vi "CRYAlignment Harmonic Orders.vi"(10 "Harmonics Orders In":dbl[](array[numeric]), 11 "HT Option":bool[](array[boolean])) -> (3 "Harmonics Orders Out":dbl[](array[numeric]))   [LabVIEW 2013]
panel:
  # "* measurement confidence\n0. Standard Error\n1. Confidence Limits\n2. Total Noise\n\n*Harmonics\n3. Harmonics @meas.Frq\n4. Total Distortion\n5. THD [%]\n6. THD Normalized [%]\n7. THD + Noise [%]\n8. Rub & Buzz [%]\n9. Rub & Buzz Norm'd [%]\n\nIM\n10. Total IM\n11. Total IM [%]\n12. Total IM + Noise [%]\n\nDiff\n13. Total Diff\n14. Total DFD [%]\n15. Total DFD + Noise [%]"
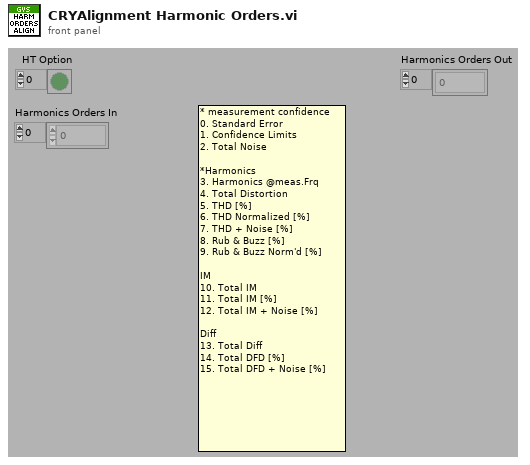
[diagram p1: front panel]
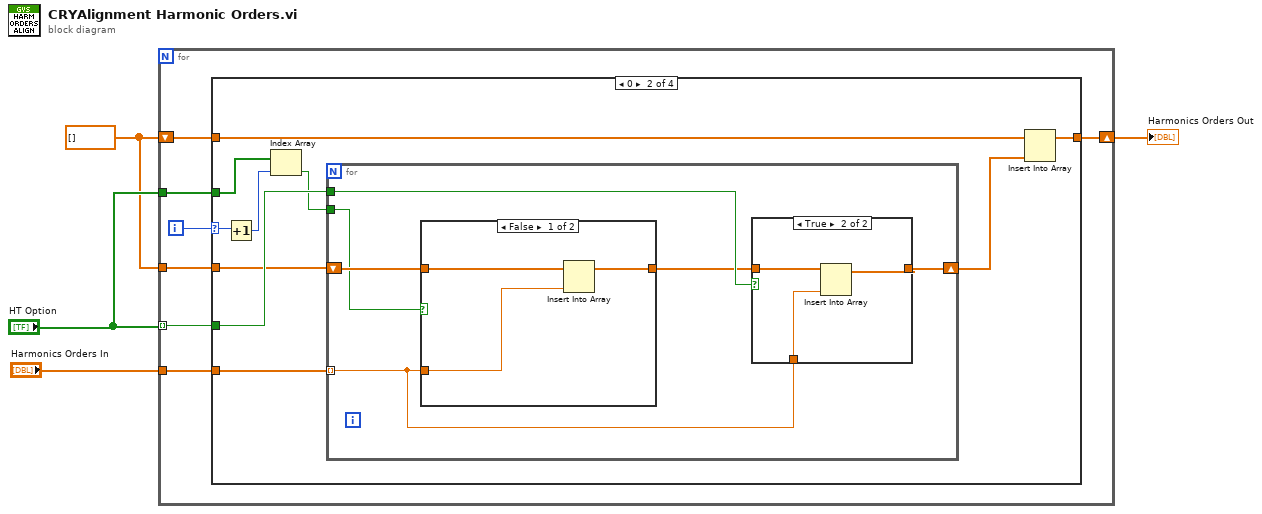
[diagram p0: block diagram]
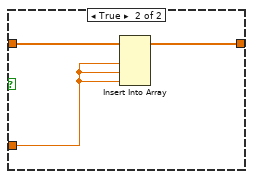
[diagram p4: hidden frame]
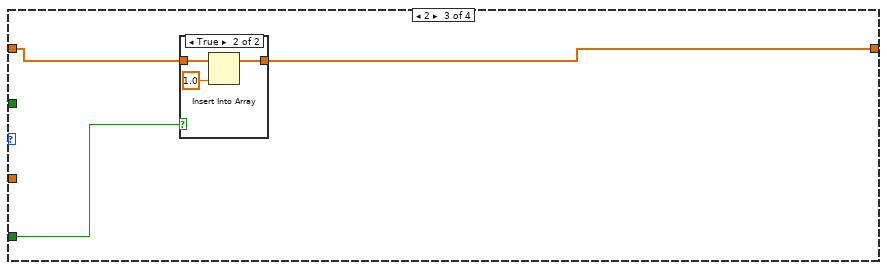
[diagram p5: hidden frame]
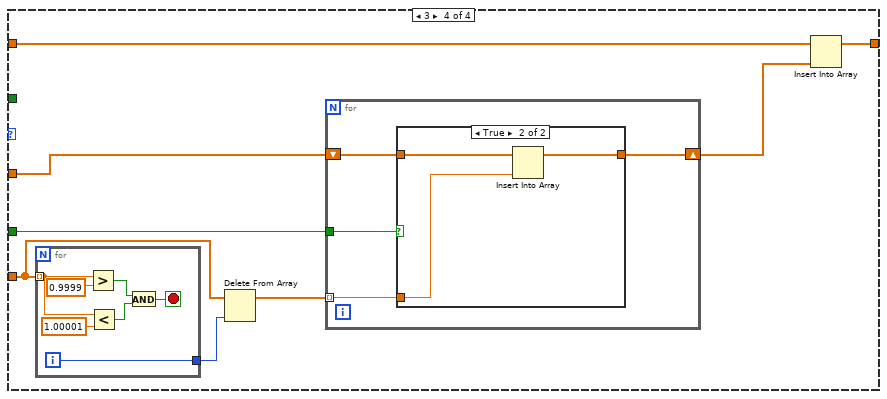
[diagram p7: hidden frame]
diagram:
  w2 = dbl[] [] ("Harmonics Orders")
  n1 = for {
    tunnel: "HT Option" -> [w9] mode=indexing
    shift-right: [w10] -> w1
    shift-left: w2 -> [w11]
    tunnel: "HT Option" -> [w7]
    tunnel: w2 -> [w6]
    tunnel: "Harmonics Orders In" -> [w5]
    i -> [w8]
    n2 = case shown="0" w8 {
      selector: w8 -> [_ w20 _ _]
      tunnel: w11 -> [w12 w16 w41 w48]
      tunnel: [w12 w17 w40 w47] -> w10
      tunnel: w9 -> [_ w22 w39 w53]
      tunnel: w7 -> [_ w21 _ _]
      tunnel: w6 -> [_ w14 _ w50]
      tunnel: w5 -> [_ w13 _ w51]
      frame Default {
      }
      frame 0 {
        n3 = Increment(x=w20) -> (x+1=w19:i32)
        n4 = Index Array(array=w21, index=w19) -> (element=w18:bool)
        n5 = for {
          tunnel: w18 -> [w26]
          shift-right: [w27] -> w15
          shift-left: w14 -> [w28]
          tunnel: w22 -> [w25]
          tunnel: w13 -> [w23] mode=indexing
          n6 = case shown="False" w26 {
            tunnel: w28 -> [w35 w38]
            tunnel: [w34 w37] -> w24
            tunnel: w23 -> [w33 w36]
            frame False {
              n7 = Insert Into Array(array=w35, new element=w33) -> (w34:dbl[])  [unwired: 1 in]
            }
            frame True {
              n8 = Insert Into Array(array=w38, new element #1=w36, new element #2=w36, new element #3=w36) -> (w37:dbl[])  [unwired: 1 in]
            }
          }
          n9 = case shown="True" w25 {
            tunnel: w24 -> [w29 w32]
            tunnel: [w29 w31] -> w27
            tunnel: w23 -> [_ w30]
            frame False {
            }
            frame True {
              n10 = Insert Into Array(array=w32, new element=w30) -> (w31:dbl[])  [unwired: 1 in]
            }
          }
        }
        n11 = Insert Into Array(array=w16, new element=w15) -> (w17:dbl[])  [unwired: 1 in]
      }
      frame 2 {
        n12 = case shown="True" w39 {
          tunnel: w41 -> [w42 w45]
          tunnel: [w42 w44] -> w40
          frame False {
          }
          frame True {
            n13 = Insert Into Array(array=w45, new element=1.0 ("new element/subarray")) -> (w44:dbl[])  [unwired: 1 in]
          }
        }
      }
      frame 3 {
        n14 = for {
          tunnel: w51 -> [w66] mode=indexing
          tunnel: [w62] -> w52
          i -> [w62]
          stop <- w63 stop-if-true
          n15 = Greater?(x=w66, y=0.9999) -> (0:w65:bool)
          n16 = Less?(x=w66, y=1.00001) -> (x < y?=w64:bool)
          n17 = And(x=w65, y=w64) -> (x .and. y?=w63:bool)
        }
        n18 = Delete From Array(array=w51, index=w52) -> (array with subset deleted=w49:dbl[])  [unwired: 1 in, 1 out]
        n19 = for {
          tunnel: w53 -> [w57]
          shift-right: [w55] -> w46
          shift-left: w50 -> [w56]
          tunnel: w49 -> [w54] mode=indexing
          n20 = case shown="True" w57 {
            tunnel: w56 -> [w58 w61]
            tunnel: [w58 w60] -> w55
            tunnel: w54 -> [_ w59]
            frame False {
            }
            frame True {
              n21 = Insert Into Array(array=w61, new element=w59) -> (w60:dbl[])  [unwired: 1 in]
            }
          }
        }
        n22 = Insert Into Array(array=w48, new element=w46) -> (w47:dbl[])  [unwired: 1 in]
      }
    }
  }
  "Harmonics Orders Out" <- w1
